vi "TestPattern.vi"() -> ()   [LabVIEW 2019]
uses:
  <vilib>/vision/NI_Vision_Development_Module.lvlib
panel:
  out "Fitted Circle":T1 {"Average SNR (dB)" format="%.2f"; "Average Strength" format="%.2f"; "Roundness (Real-World)" format="%.2f"; "Radius (Real-World)" format="%.2f"; "Center (Real-World)"."Y" format="%.2f"; "Center (Real-World)"."X" format="%.2f"; "Radius (Pixels)" format="%.2f"; "Center (Pixels)"."Y" format="%.2f"; "Center (Pixels)"."X" format="%.2f"}
  out "Circle Found":bool
  in  "ROI Descriptor":T2 {"Contours"."Type" items=["No Selection", "Point", "Line", "Rectangle", "Oval", "Polygon", "Free", "Annulus", "Unused2", "Unused3", "Broken Line", "Free Hand Line", "Rotated Rectangle"]}
  in  "File Path":path
  out "Image 2":T3(plugin-control)
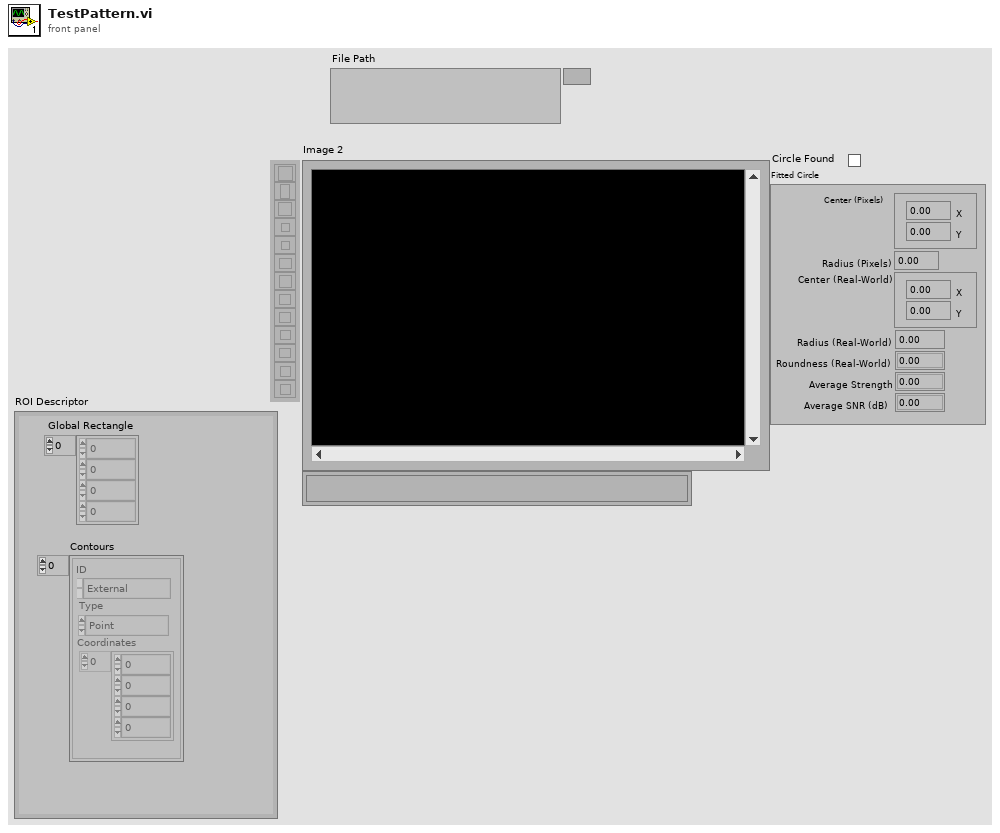
[diagram p1: front panel]
types:
  T1 = cluster{"Center (Pixels)":cluster{"X":sgl, "Y":sgl}, "Radius (Pixels)":dbl, "Center (Real-World)":cluster{"X":sgl, "Y":sgl}, "Radius (Real-World)":dbl, "Roundness (Real-World)":dbl, "Average Strength":dbl, "Average SNR (dB)":dbl}
  T2 = cluster{"Global Rectangle":i32[], "Contours":cluster{"ID":enum32{"External", "Internal"}, "Type":u32, "Coordinates":i32[]}[]}
  T3 = typedef "IMAQ Image.ctl" = refnum<image>
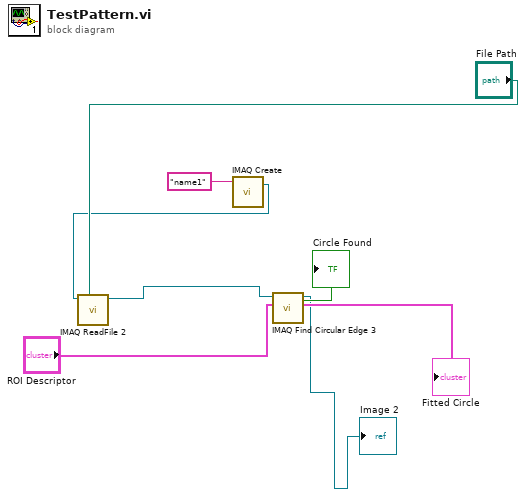
[diagram p0: block diagram]
diagram:
  n1 = call "IMAQ Create"("Image Name"="name1") -> ("New Image"=w1:T3)  [unwired: 4 in, 1 out]
  n2 = call "IMAQ ReadFile 2"("File Path"="File Path", "Image"=w1) -> ("Image Out"=w3:T3)  [unwired: 5 in, 4 out]
  n3 = call "IMAQ Find Circular Edge 3"("ROI Descriptor"="ROI Descriptor", "Image"=w3) -> ("Fitted Circle"=→"Fitted Circle":T1, "Image Out"=→"Image 2":T3, "Circle Found"=→"Circle Found":bool)  [unwired: 5 in, 2 out]
